vi "main.vi"() -> ()   [LabVIEW 2022 SP3]
uses:
  DataCluster.ctl
  a6309c79-5fe6-4af4-a42e-9fe127667a0f.vi
  b788d839-f62c-4f6b-a444-0fc034ee0148.vi
panel:
  in  "Delete":bool
  out "Progress":u8(slide)=100 scale=0.0..100.0
  in  "Download":bool
  out "Version":string="DL20 DG\nVersion 0.0.0.1"
  in  "Help":bool
  in  "File List":i32(listbox)=1
  out "Data Feed":string
  out "StatusString":string="Closing System"
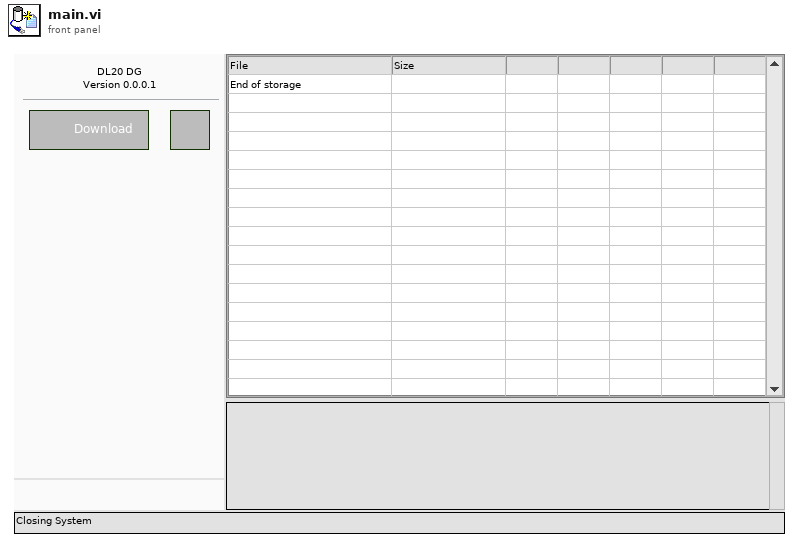
[diagram p1: front panel]
types:
  T1 = typedef "DataCluster.ctl" = cluster{"Core":cluster{"Current VI Reference":refnum<vi>, "Close Panel on Exit?":bool, "Exit":bool}, "Connections":cluster{"Arduino":cluster{"VISA":refnum<visa-resource-name>, "Data Feed":string, "Connected":bool}, "Ready":bool}, "Files":cluster{"Path":path, "Filename":string, "File List":i32, "Buffer":cluster{"Buffer":refnum<queue>, "Size":i32}, "Downloading":bool}}
  T2 = enum32{"Invalid", "Standard", "Closed", "Hidden", "Minimized", "Maximized"}
  T3 = enum32{"invalid app kind", "Development System", "Run Time System", "Student Edition", "Embedded LabVIEW", "Evaluation", "Custom"}
  T4 = cluster{"Arduino":cluster{"VISA":refnum<visa-resource-name>, "Data Feed":string, "Connected":bool}, "Ready":bool}
  T5 = enum8{"Enabled", "Disabled", "Disabled and Grayed Out"}
  T6 = cluster{"Current VI Reference":refnum<vi>, "Close Panel on Exit?":bool, "Exit":bool}
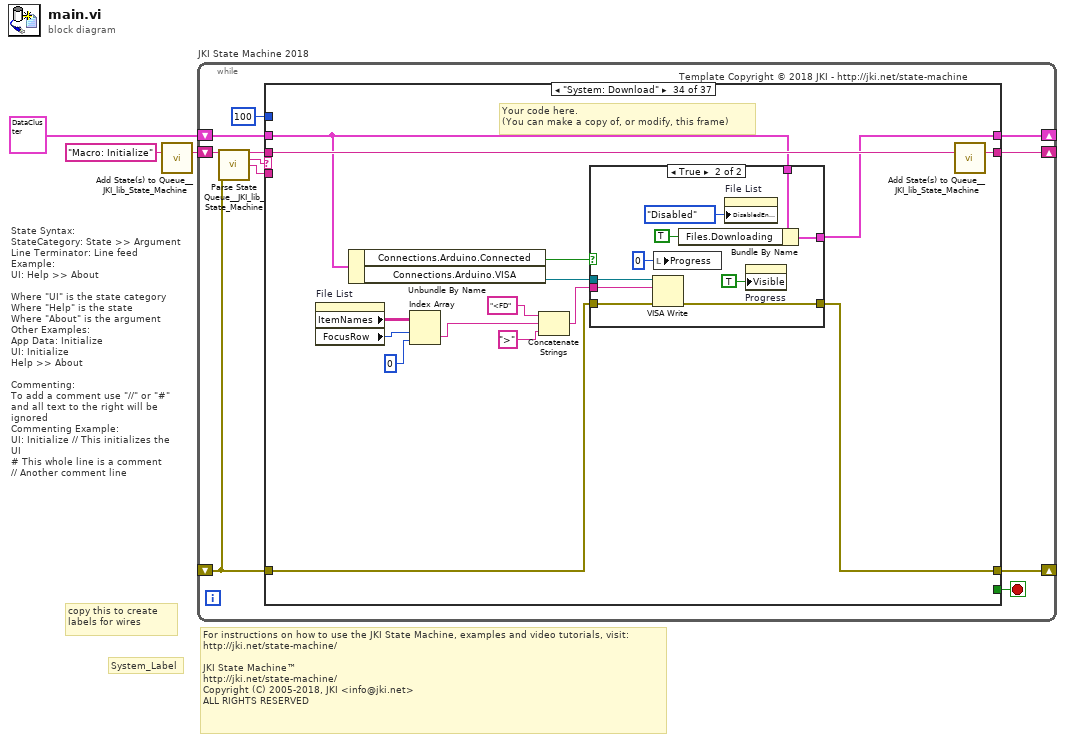
[diagram p0: block diagram]
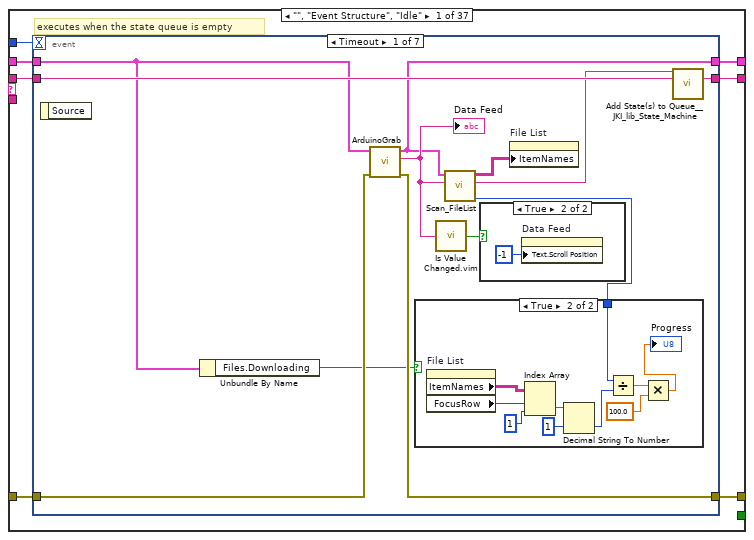
[diagram p2: hidden frame]
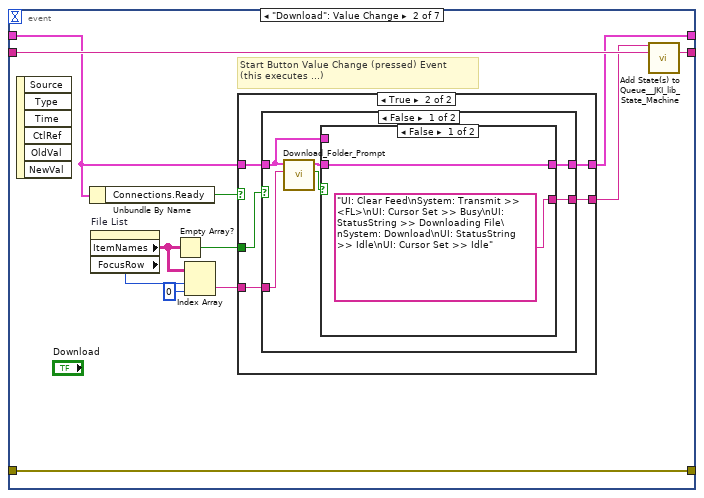
[diagram p5: hidden frame]
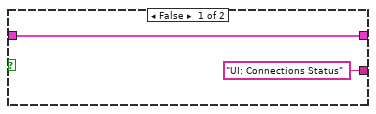
[diagram p6: hidden frame]
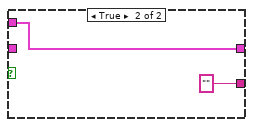
[diagram p7: hidden frame]
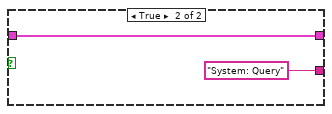
[diagram p8: hidden frame]
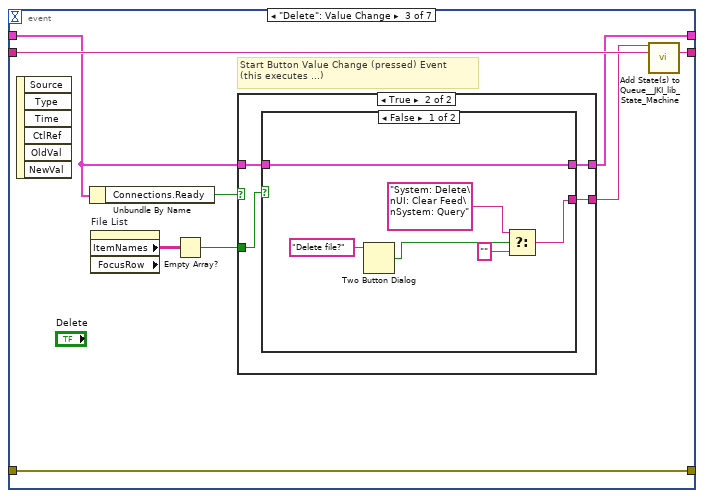
[diagram p9: hidden frame]
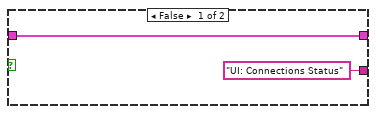
[diagram p10: hidden frame]
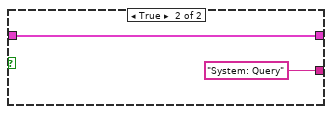
[diagram p11: hidden frame]
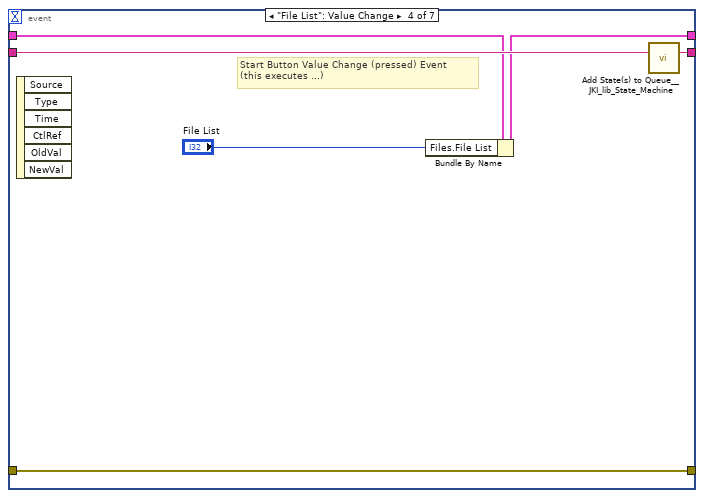
[diagram p12: hidden frame]
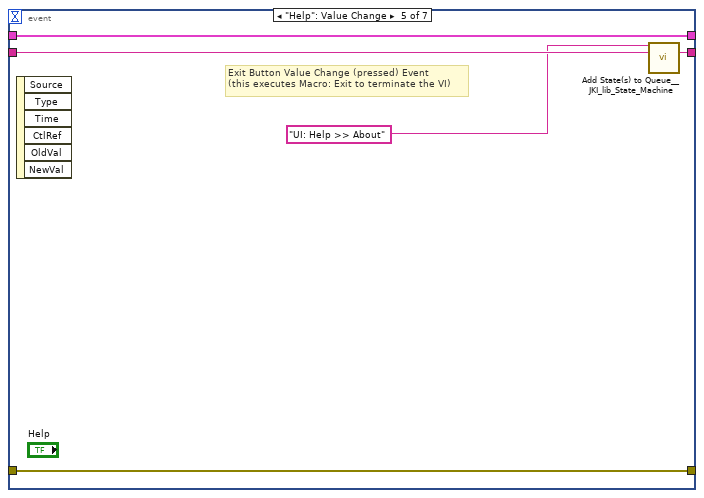
[diagram p13: hidden frame]
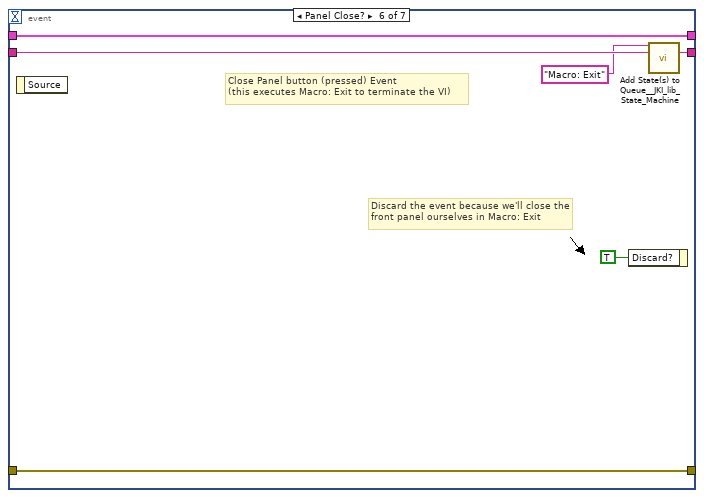
[diagram p14: hidden frame]
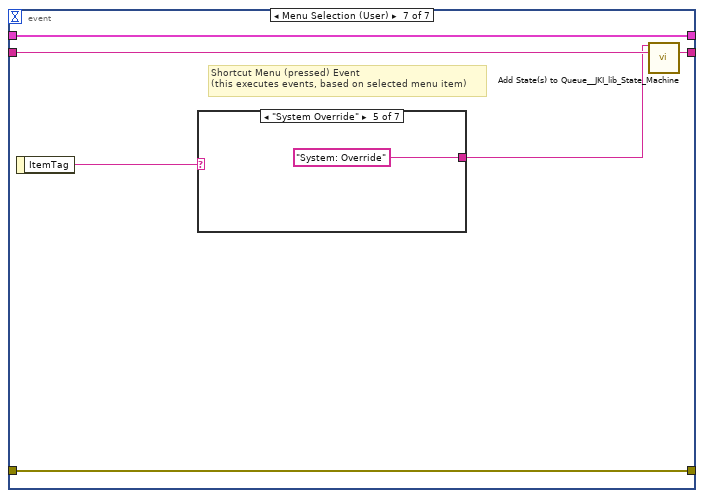
[diagram p15: hidden frame]
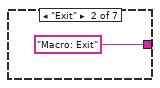
[diagram p17: hidden frame]
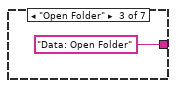
[diagram p18: hidden frame]
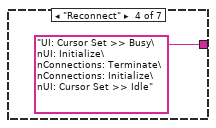
[diagram p19: hidden frame]
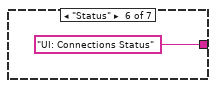
[diagram p20: hidden frame]
diagram:
  # "For instructions on how to use the JKI State Machine, examples and video tutorials, visit:\nhttp://jki.net/state-machine/\n\nJKI State Machine™\nhttp://jki.net/state-machine/\nCopyright (C) 2005-2018, JKI <info@jki.net>\nALL RIGHTS RESERVED"
  # "State Syntax:\nStateCategory: State >> Argument\nLine Terminator: Line feed\nExample:\nUI: Help >> About\n\nWhere \"UI\" is the state category\nWhere \"Help\" is the state\nWhere \"About\" is the argument\nOther Examples:\nApp Data: Initialize\nUI: Initialize\nHelp >> About\n\nCommenting:\nTo add a comment use \"//\" or \"#\" and all text to the right will be ignored\nCommenting Example:\nUI: Initialize // This initializes the UI\n# This whole line is a comment\n// Another comment line"
  # "copy this to create labels for wires"
  # "System_Label"
  n1 = call <vilib>:"Add State(s) to Queue__JKI_lib_State_Machine.vi"("State(s) in (\"\")"="Macro: Initialize") -> ("States Out"=w3:string)  [unwired: 14 in]
  n2 = while "JKI State Machine 2018" {
    shift-right: [w4] -> _
    shift-left: T1 {"Core"={"Current VI Reference"=refnum, "Close Panel on Exit?"=FALSE, "Exit"=FALSE}, "Connections"={"Arduino"={"VISA"="", "Data Feed"="", "Connected"=FALSE}, "Ready"=FALSE}, "Files"={"Path"=path "", "Filename"="", "File List"=0, "Buffer"={"Buffer"=refnum, "Size"=0}, "Downloading"=FALSE}} ("DataCluster") -> [w7]
    shift-right: [w10] -> _
    shift-left: _ -> [w5]
    shift-right: [w9] -> _
    shift-left: w3 -> [w11]
    stop <- w8 stop-if-true
    # "Template Copyright © 2018 JKI - http://jki.net/state-machine"
    n3 = call <vilib>:"Parse State Queue__JKI_lib_State_Machine.vi"("State Queue"=w11, "Error In (no error)"=w5) -> ("Remaining States"=w13:string, "Current State"=w14:string, "Arguments"=w12:string)  [unwired: 11 in]
    n4 = case shown="\"System: Download\"" w14 {
      selector: w14 -> [_ _ w132 _ _ _ _ _ _ _ _ _ _ _ _ _ _ _ _ _ _ _ _ _ _ _ _ _ _ _ _ _ _ _ _ _ _]
      tunnel: w13 -> [w21 w131 w136 w155 w161 w168 w172 w181 w188 w192 w199 w208 w212 w217 w225 w230 w238 w253 w265 w275 w285 w290 w295 w304 w313 w329 w340 w409 w414 w425 w429 w437 w450 w470 w498 w516 w520]
      tunnel: w12 -> [_ _ _ _ _ _ _ _ _ _ _ _ _ _ _ _ _ _ _ _ _ w286 w291 _ w309 w324 w334 _ _ _ _ w431 _ _ _ _ _]
      tunnel: w7 -> [w19 w128 w134 w148 w158 w164 w169 _ w185 w189 w196 w201 w209 w214 w221 w227 w234 w249 w262 w273 w283 w288 w293 w301 w311 w327 w336 w406 w411 w422 w426 w435 w448 w456 w483 w509 w517]
      tunnel: [w18 w129 w138 w152 errorcluster {"status"=FALSE, "code"=0, "source"=""} ("error out") w166 w170 w174 w182 w190 w193 w202 w210 w215 w222 w228 w231 w251 w263 w272 w282 w287 w292 w302 w310 w325 w337 w407 w412 w423 w427 w430 w444 w465 w493 w507 w518] -> w10
      tunnel: w5 -> [w17 w129 w137 w152 w157 w166 w170 w175 w184 w190 w194 w203 w210 w215 w223 w228 w232 w251 w263 w272 w282 w287 w292 w302 w310 w326 w338 w407 w412 w423 w427 w432 w445 w466 w494 w508 w518]
      tunnel: [w20 w130 w135 w154 w160 w167 w171 w180 w187 w191 w198 w207 w211 w216 w224 w229 w237 w252 w264 w274 w284 w289 w294 w303 w312 w328 w339 w408 w413 w424 w428 w436 w449 w469 w497 w515 w519] -> w9
      tunnel: [_ _ _ _ _ TRUE _ _ _ _ _ _ _ _ _ _ _ _ _ _ _ _ _ _ _ _ _ _ _ _ _ _ _ _ _ _ _] -> w8
      tunnel: [w16 w128 w134 w153 w158 w162 w169 w179 w185 w189 w196 w201 w209 w214 w220 w227 w233 w248 w262 w273 w281 w288 w293 w301 w311 w327 w336 w406 w411 w422 w426 w435 w448 w457 w483 w514 w517] -> w4
      tunnel: 100 ("Timeout") -> [w15 _ _ _ _ _ _ _ _ _ _ _ _ _ _ _ _ _ _ _ _ _ _ _ _ _ _ _ _ _ _ _ _ _ _ _ _]
      frame "", "Event Structure", "Idle" {
        # "executes when the state queue is empty"
        n5 = event shown="[0] Timeout" {
          selector: _ -> [_ _ _ _ _ _ _]
          dyn-events: _ -> [_ _ _ _ _ _ _]
          timeout: w15 -> [_ _ _ _ _ _ _]
          tunnel: w21 -> [w33 w56 w84 w104 w109 w115 w121]
          tunnel: [w32 w55 w83 w103 w108 w114 w120] -> w20
          tunnel: w19 -> [w25 w50 w78 w101 w106 w112 w118]
          tunnel: [w30 w54 w82 w102 w107 w113 w119] -> w18
          tunnel: w17 -> [w31 w54 w82 w102 w107 w113 w119]
          tunnel: [w22 w49 w77 w100 w106 w112 w118] -> w16
          event Timeout {
            n6 = event-data() -> ()  [unwired: 1 in, 1 out]
            n7 = Unbundle By Name(w25) -> ("Files.Downloading"=w24:bool)
            n8 = call "ArduinoGrab.vi"("error in (no error)"=w31, "DataCluster"=w25) -> ("error out"=w30:errorcluster, "read buffer out"=w23:string, "DataCluster out"=w22:T1)  [unwired: 6 in, 1 out]
            "Data Feed" <- w23
            n9 = call "Is Value Changed.vim"("value"=w23) -> ("changed or first call?"=w28:bool)
            n10 = call "Scan_FileList.vi"("Data Feed"=w23, "DataCluster"=w22) -> ("Downloaded bytes"=w27:i32, "state out"=w26:string, "Sorted Files"=w29:string[][])  [unwired: 7 in]
            n11 = case shown="True" w24 {
              tunnel: w27 -> [_ w35]
              frame False {
              }
              frame True {
                n12 = property on="File List" class="MCListbox (strict)"() -> ("ItemNames"=w43:string[][], "FocusRow"=w42:i32)  [unwired: 2 in, 2 out]
                n13 = Index Array(array=w43, index (row)=w42, index (col)=1 ("disabled index (col)")) -> (element=w40:string)
                n14 = Decimal String To Number(string=w40, offset=1) -> (number=w39:i32)  [unwired: 1 in, 1 out]
                n15 = Divide(x=w35, y=w39) -> (x/y=w38:dbl)
                n16 = Multiply(x=w38, y=100.0) -> (x*y=→"Progress":dbl)
              }
            }
            n17 = case shown="True" w28 {
              frame False {
              }
              frame True {
                n18 = property on="Data Feed" class="Str"("Text.Scroll Position"=-1) -> ()  [unwired: 2 in, 2 out]
              }
            }
            n19 = property on="File List" class="MCListbox (strict)"("ItemNames"=w29) -> ()  [unwired: 2 in, 2 out]
            n20 = call <vilib>:"Add State(s) to Queue__JKI_lib_State_Machine.vi"("State(s) in Front (\"\")"=w26, "State(s) in (\"\")"=w33) -> ("States Out"=w32:string)  [unwired: 13 in]
          }
          event "Download": Value Change {
            # "Start Button Value Change (pressed) Event\n(this executes ...)"
            n21 = event-data() -> ()  [unwired: 1 in, 6 out]
            n22 = Unbundle By Name(w50) -> ("Connections.Ready"=w52:bool)
            n23 = property on="File List" class="MCListbox (strict)"() -> ("ItemNames"=w48:string[][], "FocusRow"=w47:i32)  [unwired: 2 in, 2 out]
            n24 = Empty Array?(array=w48) -> (empty?=w51:bool)
            n25 = Index Array(array=w48, index (row)=w47, index (col)=0 ("disabled index (col)")) -> (element=w45:string)
            n26 = case shown="True" w52 {
              tunnel: ["UI: Connections Status" ("State(s) in Front (\"\")") w63] -> w53
              tunnel: w51 -> [_ w62]
              tunnel: w50 -> [w57 w61]
              tunnel: [w57 w60] -> w49
              tunnel: w45 -> [_ w59]
              frame False {
              }
              frame True {
                n27 = case shown="False" w62 {
                  tunnel: [w69 "System: Query" ("State(s) in Front (\"\")")] -> w63
                  tunnel: w61 -> [w65 w74]
                  tunnel: [w66 w74] -> w60
                  tunnel: w59 -> [w64 _]
                  frame False {
                    n28 = call "Download_Folder_Prompt.vi"("default name"=w64, "DataCluster"=w65) -> ("cancled?"=w68:bool, "DataCluster out"=w67:T1)  [unwired: 8 in]
                    n29 = case shown="False" w68 {
                      tunnel: ["UI: Clear Feed\nSystem: Transmit >> <FL>\nUI: Cursor Set >> Busy\nUI: StatusString >> Downloading File\nSystem: Download\nUI: StatusString >> Idle\nUI: Cursor Set >> Idle" ("State(s) in Front (\"\")") "" ("State(s) in Front (\"\")")] -> w69
                      tunnel: [w70 w73] -> w66
                      tunnel: w67 -> [w70 _]
                      tunnel: w65 -> [_ w73]
                      frame False {
                      }
                      frame True {
                      }
                    }
                  }
                  frame True {
                  }
                }
              }
            }
            n30 = call <vilib>:"Add State(s) to Queue__JKI_lib_State_Machine.vi"("State(s) in Front (\"\")"=w53, "State(s) in (\"\")"=w56) -> ("States Out"=w55:string)  [unwired: 13 in]
          }
          event "Delete": Value Change {
            # "Start Button Value Change (pressed) Event\n(this executes ...)"
            n31 = event-data() -> ()  [unwired: 1 in, 6 out]
            n32 = Unbundle By Name(w78) -> ("Connections.Ready"=w80:bool)
            n33 = property on="File List" class="MCListbox (strict)" props=["ItemNames", "FocusRow"]() -> ("ItemNames"=w76:string[][])  [unwired: 2 in, 3 out]
            n34 = Empty Array?(array=w76) -> (empty?=w79:bool)
            n35 = case shown="True" w80 {
              tunnel: ["UI: Connections Status" ("State(s) in Front (\"\")") w90] -> w81
              tunnel: w79 -> [_ w89]
              tunnel: w78 -> [w85 w88]
              tunnel: [w85 w87] -> w77
              frame False {
              }
              frame True {
                n36 = case shown="False" w89 {
                  tunnel: [w92 "System: Query" ("State(s) in Front (\"\")")] -> w90
                  tunnel: w88 -> [w96 w97]
                  tunnel: [w96 w97] -> w87
                  frame False {
                    n37 = Two Button Dialog(message="Delete file?") -> (T button?=w94:bool)  [unwired: 2 in]
                    n38 = Select(t="System: Delete\nUI: Clear Feed\nSystem: Query" ("State(s) in Front (\"\")"), s=w94, f="") -> (s? t:f=w92:string)
                  }
                  frame True {
                  }
                }
              }
            }
            n39 = call <vilib>:"Add State(s) to Queue__JKI_lib_State_Machine.vi"("State(s) in Front (\"\")"=w81, "State(s) in (\"\")"=w84) -> ("States Out"=w83:string)  [unwired: 13 in]
          }
          event "File List": Value Change {
            # "Start Button Value Change (pressed) Event\n(this executes ...)"
            n40 = event-data() -> ()  [unwired: 1 in, 6 out]
            n41 = Bundle By Name(cluster=w101, "Files.File List"="File List") -> (w100:T1)
            n42 = call <vilib>:"Add State(s) to Queue__JKI_lib_State_Machine.vi"("State(s) in (\"\")"=w104) -> ("States Out"=w103:string)  [unwired: 14 in]
          }
          event "Help": Value Change {
            # "Exit Button Value Change (pressed) Event\n(this executes Macro: Exit to terminate the VI)"
            n43 = event-data() -> ()  [unwired: 1 in, 6 out]
            n44 = call <vilib>:"Add State(s) to Queue__JKI_lib_State_Machine.vi"("State(s) in Front (\"\")"="UI: Help >> About" ("State(s) in Front (\"\")"), "State(s) in (\"\")"=w109) -> ("States Out"=w108:string)  [unwired: 13 in]
          }
          event Panel Close? {
            # "Discard the event because we'll close the front panel ourselves in Macro: Exit"
            # "Close Panel button (pressed) Event\n(this executes Macro: Exit to terminate the VI)"
            n45 = event-data() -> ()  [unwired: 1 in, 1 out]
            n46 = event-data("Discard?"=TRUE) -> ()  [unwired: 1 in, 1 out]
            n47 = call <vilib>:"Add State(s) to Queue__JKI_lib_State_Machine.vi"("State(s) in Front (\"\")"="Macro: Exit", "State(s) in (\"\")"=w115) -> ("States Out"=w114:string)  [unwired: 13 in]
          }
          event Menu Selection (User) {
            # "Shortcut Menu (pressed) Event\n(this executes events, based on selected menu item)"
            n48 = event-data() -> ("ItemTag"=w117:string)  [unwired: 1 in]
            n49 = case shown="\"System Override\"" w117 {
              tunnel: [_ "Macro: Exit" "Data: Open Folder" "UI: Cursor Set >> Busy\nUI: Initialize\nConnections: Terminate\nConnections: Initialize\nUI: Cursor Set >> Idle" "System: Override" "UI: Connections Status" "UI: Clear Feed\nSystem: Query"] -> w116
              frame "False", Default {
              }
              frame "Exit" {
              }
              frame "Open Folder" {
              }
              frame "Reconnect" {
              }
              frame "System Override" {
              }
              frame "Status" {
              }
              frame "Requery" {
              }
            }
            n50 = call <vilib>:"Add State(s) to Queue__JKI_lib_State_Machine.vi"("State(s) in Front (\"\")"=w116, "State(s) in (\"\")"=w121) -> ("States Out"=w120:string)  [unwired: 13 in]
          }
        }
      }
      frame "---------- Core ----------" {
        # "Do not put any code in this frame.\n(it is a separator no-op)"
        n51 = call <vilib>:"Add State(s) to Queue__JKI_lib_State_Machine.vi"("State(s) in (\"\")"=w131) -> ("States Out"=w130:string)  [unwired: 14 in]
      }
      frame Default {
        w141 = 42 items=["No error", "Argument error", "Memory is full", "Out of zone", "End of file", "File already open", "Generic file I/O error", "File not found", "File permission error", "Disk is full", "Duplicate path", "Too many files open", "System feature not enabled", "Resource file not found", "Cannot add resource", "Resource not found", "Image not found", "Image memory error", "Pen does not exist", "Config type invalid", "Config token not found", "Config parse error", "Config memory error", "Bad external code format", "Bad external code offset", "External code not present", "Null window", "Destroy window error", "Null menu", "Print aborted", "Bad print record", "Print driver error", "Windows error during printing", "Memory error during printing", "Print dialog error", "Generic print error", "Invalid device refnum", "Device not found", "Device parameter error", "Device unit error", "Cannot open device", "Device call aborted", "Generic error", "Cancelled by user", "Object ID too low", "Object ID too high", "Object not in heap", "Unknown heap", "Unknown object (invalid DefProc)", "Unknown object (DefProc not in table)", "Message out of range", "Invalid (null) method", "Unknown message", "Manager call not supported", "Bad address", "Network operation in progress", "Network operation timed out", "Connection is busy", "Network attribute not supported", "Network error", "Address in use", "System out of memory", "Connection aborted", "Connection refused", "Not connected", "Already connected", "Connection closed", "Initialization error (interapplication manager)", "Bad occurrence", "Wait on unbound occurrence handler", "Occurrence queue overflow", "Datalog type conflict", "Unused", "Unrecognized type (interapplication manager)", "Memory corrupt", "Failed to make temporary DLL", "Old CIN version", "Drag socket not found", "Failed to load drop-object", "Failed to register OLE object", "Failed to release OLE object", "Format specifier type mismatch", "Unknown format specifier", "Too few format specifiers", "Too many format specifiers", "Scan failed", "Newer CIN version", "Error converting to variant", "Runtime menu error", "Password tampered", "Variant attribute not found", "Incompatible variant data type", "Event data is not available", "Event Store is not present", "Occurrence is not found", "Event Queue is not created", "Event info is not available", "Refnum passed is NULL", "Error retrieving Class GUID", "Error retrieving CoClass GUID", "Error retrieving TypeLib GUID.", "Bad built application magic bytes.", "Specific driver is different from the specific driver associated with the Logical Name.", "There is no session opened to the class driver.", "Max Error", "MAX - Error with config objects", "MAX - Error loading configuration", "MAX - Group not supported"]
        # "Current State"
        # "Do not delete, rename, or modify this frame.\n(this is used to capture unhandled states and typos)"
        # "Handle mistyped state name (developer tool)"
        n52 = Format Into String(format string="Software Exception: Unhandled State \"%s\"." ("message"), error in=w137, w132) -> (resulting string=w140:string, error out=w139:errorcluster)  [unwired: 1 in]
        n53 = call <vilib>:"Error Cluster From Error Code.vi"("show call chain? (False)"=TRUE, "error in (no error)"=w139, "error message (\"\")"=w140, "error code (0)"=w141) -> ("error out"=w138:errorcluster)  [unwired: 5 in]
        n54 = call <vilib>:"Add State(s) to Queue__JKI_lib_State_Machine.vi"("State(s) in (\"\")"=w136) -> ("States Out"=w135:string)  [unwired: 14 in]
      }
      frame "Initialize Core Data" {
        # "Do not delete, rename, or modify this frame.\n(this is used to determine panel behavior on exit)"
        # "originally closed?"
        # "exe?"
        # "If panel starts closed or is an EXE, then close it when we exit"
        n55 = property class="VI"() -> ("FP.State"=w145:T2)  [unwired: 2 in, 2 out]
        n56 = property class="App"() -> ("App.Kind"=w151:T3)  [unwired: 2 in, 2 out]
        n57 = control-ref of="Current VI Reference"() -> (w146:refnum<vi>)
        n58 = Equal?(x=w145, y=T2."Closed" ("Front Panel Window:State")) -> (x = y?=w143:bool)
        n59 = Equal?(x=w151, y=T3."Run Time System" ("Application:Kind")) -> (x = y?=w149:bool)
        n60 = Or(x=w143, y=w149) -> (x .or. y?=w147:bool)
        n61 = Bundle By Name(cluster=w148, "Core.Current VI Reference"=w146, "Core.Close Panel on Exit?"=w147) -> (w153:T1)
        n62 = call <vilib>:"Add State(s) to Queue__JKI_lib_State_Machine.vi"("State(s) in (\"\")"=w155) -> ("States Out"=w154:string)  [unwired: 14 in]
      }
      frame "Error Handler" {
        # "Unhandled Error -- Display it"
        # "Handle any errors here.\nYou can also output any states to clean-up after errors occur"
        # "Clear error"
        n63 = call <vilib>:"General Error Handler.vi"("error in (no error)"=w157) -> ()  [unwired: 10 in, 5 out]
        n64 = call <vilib>:"Add State(s) to Queue__JKI_lib_State_Machine.vi"("State(s) in Front (\"\")"="/* Post Error States", "State(s) in (\"\")"=w161) -> ("States Out"=w160:string)  [unwired: 13 in]
      }
      frame "Exit" {
        # "Do not put any code in this frame.\n(No errors that occur here will be handled.)"
        n65 = Bundle By Name(cluster=w164, "Core.Exit"=TRUE) -> (w162:T1)
        n66 = call <vilib>:"Add State(s) to Queue__JKI_lib_State_Machine.vi"("State(s) in (\"\")"=w168) -> ("States Out"=w167:string)  [unwired: 14 in]
      }
      frame "---------- Data ----------" {
        # "Do not put any code in this frame.\n(It is a separator no-op. You can make a copy of this frame to create a new Data frame)"
        n67 = call <vilib>:"Add State(s) to Queue__JKI_lib_State_Machine.vi"("State(s) in (\"\")"=w172) -> ("States Out"=w171:string)  [unwired: 14 in]
      }
      frame "Data: Initialize" {
        w178 = T6 {"Current VI Reference"=refnum, "Close Panel on Exit?"=FALSE, "Exit"=FALSE}  # Core
        # "Initialize the shift-register data, here.\n(data names are defined by what you wire into the bundle function)"
        n68 = call "Settings_Load.vi"("error in"=w175) -> ("error out"=w176:errorcluster, "DataCluster out"=w177:T1)  [unwired: 9 in]
        n69 = call "Settings_Save.vi"("error in"=w176, "DataCluster"=w177) -> ("error out"=w174:errorcluster)  [unwired: 9 in]
        n70 = Bundle By Name(cluster=w177, "Core"=w178, "Connections"=T4 {"Arduino"={"VISA"="", "Data Feed"="", "Connected"=FALSE}, "Ready"=FALSE}) -> (w179:T1)
        n71 = call <vilib>:"Add State(s) to Queue__JKI_lib_State_Machine.vi"("State(s) in (\"\")"=w181) -> ("States Out"=w180:string)  [unwired: 14 in]
      }
      frame "Data: Cleanup" {
        # "Cleanup any data and references, here.\n(this is called automatically, by the Macro: Exit)"
        n72 = Unbundle By Name(w185) -> ("Core.Current VI Reference"=w186:refnum<vi>)
        n73 = call "Settings_Save.vi"("error in"=w184, "DataCluster"=w185) -> ("error out"=w183:errorcluster)  [unwired: 9 in]
        n74 = Close Reference(reference=w186, error in (no error)=w183) -> (error out=w182:errorcluster)
        n75 = call <vilib>:"Add State(s) to Queue__JKI_lib_State_Machine.vi"("State(s) in (\"\")"=w188) -> ("States Out"=w187:string)  [unwired: 14 in]
      }
      frame "Data: Options" {
        # "Access Data Setup here.\n(this is called automatically, by the Settings Event Run time menu)"
        n76 = call <vilib>:"Add State(s) to Queue__JKI_lib_State_Machine.vi"("State(s) in (\"\")"=w192) -> ("States Out"=w191:string)  [unwired: 14 in]
      }
      frame "Data: Files Unlock" {
        # "Unluck Data filehere.\n(this is called automatically, by the Settings Event Run time menu)"
        n77 = Unbundle By Name(w196) -> ("Files.Path"=w195:path)
        n78 = Set Permissions(7:i16 448 ("permissions"), 8:w194, 11:w195) -> (0:w193:errorcluster)  [unwired: 2 in, 1 out]
        n79 = call <vilib>:"Add State(s) to Queue__JKI_lib_State_Machine.vi"("State(s) in (\"\")"=w199) -> ("States Out"=w198:string)  [unwired: 14 in]
      }
      frame "Data: Open Folder" {
        # "Access Data Setup here.\n(this is called automatically, by the Settings Event Run time menu)"
        n80 = Unbundle By Name(w201) -> ("Files.Path"=w200:path)
        n81 = Format Into String(format string="cmd /c explorer.exe \"%s\"", w200) -> (resulting string=w205:string)  [unwired: 2 in, 1 out]
        n82 = call <vilib>:"System Exec.vi"("run minimized? (F)"=TRUE, "error in (no error)"=w203, "command line"=w205) -> ("error out"=w202:errorcluster)  [unwired: 5 in, 3 out]
        n83 = call <vilib>:"Add State(s) to Queue__JKI_lib_State_Machine.vi"("State(s) in (\"\")"=w208) -> ("States Out"=w207:string)  [unwired: 14 in]
      }
      frame "---------- Connections ----------" {
        # "Do not put any code in this frame.\n(It is a separator no-op. You can make a copy of this frame to create a new Data frame)"
        n84 = call <vilib>:"Add State(s) to Queue__JKI_lib_State_Machine.vi"("State(s) in (\"\")"=w212) -> ("States Out"=w211:string)  [unwired: 14 in]
      }
      frame "Connections: Initialize" {
        # "Initialize the System Connections, here.\n(this is called automatically, by the Macro: Init)"
        n85 = call <vilib>:"Add State(s) to Queue__JKI_lib_State_Machine.vi"("State(s) in Front (\"\")"="UI: StatusString >> Connecting to System\nConnections: Initialize Arduino\nUI: StatusString >> Validating Connections\nConnections: Status" ("State(s) in Front (\"\")"), "State(s) in (\"\")"=w217) -> ("States Out"=w216:string)  [unwired: 13 in]
      }
      frame "Connections: Initialize Arduino" {
        # "Initialize the System Connections, here.\n(this is called automatically, by the Macro: Init)"
        n86 = call "ConnectionArduino.vi"("error in"=w223) -> ("error out"=w222:errorcluster, 2:"Arduino"=w218:bool, 3:"Arduino"=w219:refnum<visa-resource-name>)  [unwired: 8 in]
        n87 = Bundle By Name(cluster=w221, "Connections.Arduino.VISA"=w219, "Connections.Arduino.Connected"=w218) -> (w220:T1)
        n88 = call <vilib>:"Add State(s) to Queue__JKI_lib_State_Machine.vi"("State(s) in (\"\")"=w225) -> ("States Out"=w224:string)  [unwired: 14 in]
      }
      frame "Connections: Terminate" {
        # "Terminate connections"
        # "Terminate the System Connections, here.\n(this is called automatically, by the Macro: Exit)"
        n89 = call <vilib>:"Add State(s) to Queue__JKI_lib_State_Machine.vi"("State(s) in Front (\"\")"="UI: StatusString >> Terminating System Connection\nConnections: Terminate Arduino" ("State(s) in Front (\"\")"), "State(s) in (\"\")"=w230) -> ("States Out"=w229:string)  [unwired: 13 in]
      }
      frame "Connections: Terminate Arduino" {
        # "Terminate connection to Arduino"
        # "Terminate the System Connections, here.\n(this is called automatically, by the Macro: Exit)"
        n90 = Unbundle By Name(w234) -> ("Connections.Arduino.VISA"=w235:refnum<visa-resource-name>, "Connections.Arduino.Connected"=w236:bool)
        n91 = case shown="True" w236 {
          tunnel: w235 -> [_ w241]
          tunnel: w234 -> [w240 w246]
          tunnel: [w240 w244] -> w233
          tunnel: w232 -> [w239 w243]
          tunnel: [w239 w242] -> w231
          frame False {
          }
          frame True {
            n92 = VISA Close(VISA resource name=w241, error in (no error)=w243) -> (error out=w242:errorcluster)
            n93 = Bundle By Name(cluster=w246, "Connections.Arduino.Connected"=FALSE ("Connections.cDAQ.Connected")) -> (w244:T1)
          }
        }
        n94 = call <vilib>:"Add State(s) to Queue__JKI_lib_State_Machine.vi"("State(s) in (\"\")"=w238) -> ("States Out"=w237:string)  [unwired: 14 in]
      }
      frame "Connections: Status" {
        # "Checks Connection Status , here.\n(this is called automatically, by the Connections: Initialize)"
        n95 = Unbundle By Name(w249) -> ("Connections.Arduino.Connected"=w247:bool)
        n96 = case shown="False" w247 {
          selector: w247 -> [w254 w259]
          tunnel: ["UI: Start Button >> Error\nUI: StatusString >> Connection Error!" "UI: Start Button >> Default\nUI: StatusString >> Idle"] -> w250
          tunnel: w249 -> [w256 w260]
          tunnel: [w255 w258] -> w248
          frame False {
            n97 = Bundle By Name(cluster=w256, "Connections.Ready"=w254) -> (w255:T1)
          }
          frame True {
            n98 = Bundle By Name(cluster=w260, "Connections.Ready"=w259) -> (w258:T1)
          }
        }
        n99 = call <vilib>:"Add State(s) to Queue__JKI_lib_State_Machine.vi"("State(s) in Front (\"\")"=w250, "State(s) in (\"\")"=w253) -> ("States Out"=w252:string)  [unwired: 13 in]
      }
      frame "---------- UI ----------" {
        # "Do not put any code in this frame.\n(It is a separator no-op. You can make a copy of this frame to create a new UI frame)"
        n100 = call <vilib>:"Add State(s) to Queue__JKI_lib_State_Machine.vi"("State(s) in (\"\")"=w265) -> ("States Out"=w264:string)  [unwired: 14 in]
      }
      frame "UI: Initialize" {
        # "Initialize the User Interface, here.\n(this is called automatically, by the Macro: Init)"
        n101 = for {
          N: 50 -> [_]
          i -> [w278]
          n102 = Bundle(w278, 1) -> (w279:cluster{i32, i32})  [unwired: 1 in]
          n103 = property on="File List" class="MCListbox (strict)"("ActiveCell"=w279, "Justify"=enum16{"Left", "Center", "Right"}."Right" ("Active Cell:Cell Justification")) -> ()  [unwired: 2 in, 2 out]
        }
        n104 = property on="File List" class="MCListbox (strict)"("ItemNames"=string[][] [] ("Item Names")) -> ()  [unwired: 2 in, 2 out]
        n105 = call "Read Exe Version.vi"() -> ("String"=→"Version":string)  [unwired: 10 in, 1 out]
        n106 = property on="Progress" class="Slide (strict)"("Visible"=FALSE) -> ()  [unwired: 2 in, 2 out]
        n107 = property on="File List" class="MCListbox (strict)"("DisabledEnum"=T5."Enabled" ("Disabled")) -> ()  [unwired: 2 in, 2 out]
        n108 = call <vilib>:"Add State(s) to Queue__JKI_lib_State_Machine.vi"("State(s) in Front (\"\")"="UI: Clear Feed" ("State(s) in Front (\"\")"), "State(s) in (\"\")"=w275) -> ("States Out"=w274:string)  [unwired: 13 in]
      }
      frame "UI: Clear Feed" {
        w280 = "" ("Data Feed")
        # "Initialize the User Interface, here.\n(this is called automatically, by the Macro: Init)"
        n109 = Bundle By Name(cluster=w283, "Connections.Arduino.Data Feed"=w280) -> (w281:T1)
        n110 = local write "Data Feed"(w280) -> ()
        n111 = call <vilib>:"Add State(s) to Queue__JKI_lib_State_Machine.vi"("State(s) in (\"\")"=w285) -> ("States Out"=w284:string)  [unwired: 14 in]
      }
      frame "UI: StatusString" {
        # "Argument"
        # "Set Status String here\n(this is called takes argument and applies to Status String)"
        n112 = call <vilib>:"Add State(s) to Queue__JKI_lib_State_Machine.vi"("State(s) in (\"\")"=w290) -> ("States Out"=w289:string)  [unwired: 14 in]
        "StatusString" <- w286
      }
      frame "UI: Help" {
        # "Argument"
        # "Set Status String here\n(this is called takes argument and applies to Status String)"
        n113 = case shown="\"About\"" w291 {
          frame "False", Default {
          }
          frame "About" {
            n114 = call "Read Exe Version.vi"() -> ("String"=w296:string)  [unwired: 10 in, 1 out]
            n115 = Concatenate Strings("Drill Logger Data Grab\n\n" ("message"), w296) -> (w297:string)
            n116 = One Button Dialog(message=w297) -> ()  [unwired: 1 in, 1 out]
          }
        }
        n117 = call <vilib>:"Add State(s) to Queue__JKI_lib_State_Machine.vi"("State(s) in (\"\")"=w295) -> ("States Out"=w294:string)  [unwired: 14 in]
      }
      frame "UI: Connections Status" {
        # "Set Status String here\n(this is called takes argument and applies to Status String)"
        n118 = Unbundle By Name(w301) -> ("Connections.Arduino.Connected"=w300:bool)
        n119 = call "ConnectionStatus.vi"("Connection Status"=w300) -> ("String"=w299:string)  [unwired: 9 in, 1 out]
        n120 = call <vilib>:"Add State(s) to Queue__JKI_lib_State_Machine.vi"("State(s) in Front (\"\")"=w299, "State(s) in (\"\")"=w304) -> ("States Out"=w303:string)  [unwired: 13 in]
      }
      frame "UI: Start Button" {
        # "Argument"
        # "Set Status String here\n(this is called takes argument and applies to Status String)"
        n121 = case shown="\"Connecting\"" w309 {
          tunnel: [w314 cluster{u32, u32}[] [{1985280, 12369084}, {4367360, 4367360}, {8388608, 16711681}, {1985280, 1985280}, {1985280, 4367360}, {8388608, 16711681}] ("Colors [4]") w321] -> w306
          tunnel: [string[] ["  Error", "  Error", "  Error", "  Error"] ("Strings [4]") string[] ["Download", "Download", "Download", "Download"] ("Strings [4]") string[] ["Connecting", "Connecting", "Connecting", "Connecting"] ("Strings [4]")] -> w308
          tunnel: [T5."Enabled" ("Disabled") T5."Enabled" ("Disabled") T5."Disabled" ("Disabled")] -> w307
          tunnel: [w314 cluster{u32, u32}[] [{1985280, 12369084}, {8388608, 16711681}, {8388608, 16711681}, {8388608, 8388608}, {8388608, 8388608}, {8388608, 16711681}] ("Colors [4]") w321] -> w305
          frame "Error" {
            w314 = cluster{u32, u32}[] [{8388608, 8388608}, {4367360, 4367360}, {9342611, 9342611}, {6710891, 6710891}, {16711681, 16711680}, {16711681, 16711680}] ("Colors [4]")
          }
          frame "Default", Default {
          }
          frame "Connecting" {
            w321 = cluster{u32, u32}[] [{9342611, 9342611}, {4367360, 4367360}, {9342611, 9342611}, {6710891, 6710891}, {9342611, 9342611}, {9342611, 9342611}] ("Colors [4]")
          }
        }
        n122 = property on="Download" class="Bool"("Colors [4]"=w306, "Strings [4]"=w308, "DisabledEnum"=w307) -> ()  [unwired: 2 in, 2 out]
        n123 = property on="Delete" class="Bool"("Colors [4]"=w305, "DisabledEnum"=w307) -> ()  [unwired: 2 in, 2 out]
        n124 = call <vilib>:"Add State(s) to Queue__JKI_lib_State_Machine.vi"("State(s) in (\"\")"=w313) -> ("States Out"=w312:string)  [unwired: 14 in]
      }
      frame "UI: Cursor Set" {
        # "Argument"
        # "Set and Unset Cursor Busy.\n(Usage: \"UI: Cursor Set >> Busy|Idle\")"
        n125 = case shown="\"Idle\", Default" w324 {
          tunnel: w326 -> [w331 w333]
          tunnel: [w330 w332] -> w325
          frame "Idle", Default {
            n126 = call <vilib>:"Unset Busy.vi"("error in (no error)"=w331) -> ("error out"=w330:errorcluster)  [unwired: 10 in]
          }
          frame "Busy" {
            n127 = call <vilib>:"Set Busy.vi"("error in (no error)"=w333) -> ("error out"=w332:errorcluster)  [unwired: 9 in, 1 out]
          }
        }
        n128 = call <vilib>:"Add State(s) to Queue__JKI_lib_State_Machine.vi"("State(s) in (\"\")"=w329) -> ("States Out"=w328:string)  [unwired: 14 in]
      }
      frame "UI: Front Panel State" {
        # "Argument"
        # "Set Front Panel Open or Closed\n(Usage: \"UI: Front Panel State >> Open|Close\")"
        n129 = Unbundle By Name(w336) -> ("Core.Current VI Reference"=w335:refnum<vi>)
        n130 = case shown="\"Minimize\", \"Minimized\"" w334 {
          tunnel: w338 -> [w346 w361 w372 w385 w398]
          tunnel: [w348 w362 w374 w387 w400] -> w337
          tunnel: w335 -> [w347 w359 w373 w386 w399]
          frame "Open", "Standard", Default {
            w341 = T2."Standard" ("State")
            n131 = property class="VI"(reference=w347, error in=w346) -> (reference out=w344:refnum<vi>, error out=w345:errorcluster, "FP.State"=w343:T2)
            n132 = Not Equal?(x=w343, y=w341) -> (x != y?=w342:bool)
            n133 = case shown="True" w342 {
              tunnel: [w352 w354] -> w348
              tunnel: w345 -> [w351 w354]
              tunnel: w344 -> [w350 _]
              tunnel: w341 -> [w349 _]
              frame True {
                n134 = invoke class="VI" method="FP.Open"(reference=w350, error in=w351, "Activate"=TRUE, "State"=w349) -> (error out=w352:errorcluster)  [unwired: 1 in, 4 out]
              }
              frame False {
              }
            }
          }
          frame "Close", "Closed" {
            n135 = property class="VI"(reference=w359, error in=w361) -> (reference out=w358:refnum<vi>, error out=w360:errorcluster, "FP.State"=w356:T2)
            n136 = Not Equal?(x=w356, y=T2."Closed" ("Front Panel Window:State")) -> (x != y?=w355:bool)
            n137 = case shown="True" w355 {
              tunnel: [w363 w366] -> w362
              tunnel: w360 -> [w363 w365]
              tunnel: w358 -> [_ w364]
              frame False {
              }
              frame True {
                n138 = invoke class="VI" method="FP.Close"(reference=w364, error in=w365) -> (error out=w366:errorcluster)  [unwired: 1 in, 2 out]
              }
            }
          }
          frame "Hidden", "Hide" {
            w367 = T2."Hidden" ("State")
            n139 = property class="VI"(reference=w373, error in=w372) -> (reference out=w370:refnum<vi>, error out=w371:errorcluster, "FP.State"=w369:T2)
            n140 = Not Equal?(x=w369, y=w367) -> (x != y?=w368:bool)
            n141 = case shown="True" w368 {
              tunnel: [w378 w379] -> w374
              tunnel: w371 -> [w377 w379]
              tunnel: w370 -> [w376 _]
              tunnel: w367 -> [w375 _]
              frame True {
                n142 = invoke class="VI" method="FP.Open"(reference=w376, error in=w377, "State"=w375) -> (error out=w378:errorcluster)  [unwired: 2 in, 4 out]
              }
              frame False {
              }
            }
          }
          frame "Minimize", "Minimized" {
            w380 = T2."Minimized" ("State")
            n143 = property class="VI"(reference=w386, error in=w385) -> (reference out=w383:refnum<vi>, error out=w384:errorcluster, "FP.State"=w382:T2)
            n144 = Not Equal?(x=w382, y=w380) -> (x != y?=w381:bool)
            n145 = case shown="True" w381 {
              tunnel: [w391 w392] -> w387
              tunnel: w384 -> [w390 w392]
              tunnel: w383 -> [w389 _]
              tunnel: w380 -> [w388 _]
              frame True {
                n146 = invoke class="VI" method="FP.Open"(reference=w389, error in=w390, "State"=w388) -> (error out=w391:errorcluster)  [unwired: 2 in, 4 out]
              }
              frame False {
              }
            }
          }
          frame "Maximize", "Maximized" {
            w393 = T2."Maximized" ("State")
            n147 = property class="VI"(reference=w399, error in=w398) -> (reference out=w396:refnum<vi>, error out=w397:errorcluster, "FP.State"=w395:T2)
            n148 = Not Equal?(x=w395, y=w393) -> (x != y?=w394:bool)
            n149 = case shown="True" w394 {
              tunnel: [w404 w405] -> w400
              tunnel: w397 -> [w403 w405]
              tunnel: w396 -> [w402 _]
              tunnel: w393 -> [w401 _]
              frame True {
                n150 = invoke class="VI" method="FP.Open"(reference=w402, error in=w403, "State"=w401) -> (error out=w404:errorcluster)  [unwired: 2 in, 4 out]
              }
              frame False {
              }
            }
          }
        }
        n151 = call <vilib>:"Add State(s) to Queue__JKI_lib_State_Machine.vi"("State(s) in (\"\")"=w340) -> ("States Out"=w339:string)  [unwired: 14 in]
      }
      frame "---------- Macro ----------" {
        # "Do not put any code in this frame.\n(It is a separator no-op. You can make a copy of this frame to create a new Macro frame)"
        n152 = call <vilib>:"Add State(s) to Queue__JKI_lib_State_Machine.vi"("State(s) in (\"\")"=w409) -> ("States Out"=w408:string)  [unwired: 14 in]
      }
      frame "Macro: Initialize" {
        w410 = "UI: StatusString >> Initializing...\nUI: Cursor Set >> Busy\nUI: Start Button >> Connecting\nUI: StatusString >> Initializing Data\nData: Initialize\nUI: StatusString >> Initializing Core Data\nInitialize Core Data\nUI: StatusString >> Initializing User Interface\nUI: Initialize\nUI: StatusString >> Initializing Connections\nConnections: Initialize\nUI: StatusString >> Query Data\nSystem: Query\nConnections: Status\nUI: Front Panel State >> Open\nUI: Cursor Set >> Idle"  # UI: StatusString >> Initializing... UI: Cursor Set >> Busy UI: Start Button >> Connecting UI: StatusString >> Initializing Data Data: Initialize UI: StatusString >> Initializing Core Data Initialize Core Data UI: StatusString >> Initializing User Interface UI: Initialize UI: StatusString >> Initializing Connections Connections: Initialize UI: StatusString >> Query Data System: Query Connections: Status UI: Front Panel State >> Open UI: Cursor Set >> Idle
        # "Initialization Macro\n(This is called once, when the VI starts)"
        n153 = call <vilib>:"Add State(s) to Queue__JKI_lib_State_Machine.vi"("State(s) in Front (\"\")"=w410, "State(s) in (\"\")"=w414) -> ("States Out"=w413:string)  [unwired: 13 in]
      }
      frame "Macro: Exit" {
        # "Exit Macro\n(This is called once, when the VI exits)"
        n154 = Unbundle By Name(w422) -> ("Core.Close Panel on Exit?"=w421:bool)
        n155 = Select(t="UI: Front Panel State >> Close", s=w421, f="") -> (s? t:f=w418:string)
        n156 = call <vilib>:"Add State(s) to Queue__JKI_lib_State_Machine.vi"("State(s) in Front (\"\")"="UI: StatusString >> Closing System... Terminating Connections\nConnections: Terminate\nUI: StatusString >> Closing System... Data Cleanup\nData: Cleanup\nUI: StatusString >> Closing System" ("State(s) in Front (\"\")"), "State(s) in (\"\")"=w418, "State(s) at Back (\"\")"="Exit") -> ("States Out"=w417:string)  [unwired: 12 in]
        n157 = call <vilib>:"Add State(s) to Queue__JKI_lib_State_Machine.vi"("State(s) in Front (\"\")"=w417, "State(s) in (\"\")"=w425) -> ("States Out"=w424:string)  [unwired: 13 in]
      }
      frame "---------- System ----------" {
        # "Template Separator\n(You can make a copy of, or modify, this frame)"
        n158 = call <vilib>:"Add State(s) to Queue__JKI_lib_State_Machine.vi"("State(s) in (\"\")"=w429) -> ("States Out"=w428:string)  [unwired: 14 in]
      }
      frame "System: Transmit" {
        # "Your code here.\n(You can make a copy of, or modify, this frame)"
        n159 = Unbundle By Name(w435) -> ("Connections.Arduino.Connected"=w434:bool, "Connections.Arduino.VISA"=w433:refnum<visa-resource-name>)
        n160 = case shown="True" w434 {
          tunnel: w433 -> [_ w442]
          tunnel: w432 -> [w438 w441]
          tunnel: [w438 w440] -> w430
          tunnel: w431 -> [_ w439]
          frame False {
          }
          frame True {
            n161 = VISA Write(VISA resource name=w442, write buffer=w439, error in (no error)=w441) -> (error out=w440:errorcluster)  [unwired: 2 out]
          }
        }
        n162 = call <vilib>:"Add State(s) to Queue__JKI_lib_State_Machine.vi"("State(s) in (\"\")"=w437) -> ("States Out"=w436:string)  [unwired: 14 in]
      }
      frame "System: Query" {
        # "Your code here.\n(You can make a copy of, or modify, this frame)"
        n163 = Unbundle By Name(w448) -> ("Connections.Arduino.Connected"=w447:bool, "Connections.Arduino.VISA"=w446:refnum<visa-resource-name>)
        n164 = case shown="True" w447 {
          tunnel: w446 -> [_ w455]
          tunnel: w445 -> [w451 w454]
          tunnel: [w451 w453] -> w444
          tunnel: "<FL>" ("Arguments") -> [_ w452]
          frame False {
          }
          frame True {
            n165 = VISA Write(VISA resource name=w455, write buffer=w452, error in (no error)=w454) -> (error out=w453:errorcluster)  [unwired: 2 out]
          }
        }
        n166 = call <vilib>:"Add State(s) to Queue__JKI_lib_State_Machine.vi"("State(s) in (\"\")"=w450) -> ("States Out"=w449:string)  [unwired: 14 in]
      }
      frame "System: Download" {
        # "Your code here.\n(You can make a copy of, or modify, this frame)"
        n167 = property on="File List" class="MCListbox (strict)"() -> ("ItemNames"=w460:string[][], "FocusRow"=w459:i32)  [unwired: 2 in, 2 out]
        n168 = Unbundle By Name(w456) -> ("Connections.Arduino.Connected"=w468:bool, "Connections.Arduino.VISA"=w467:refnum<visa-resource-name>)
        n169 = Index Array(array=w460, index (row)=w459, index (col)=0 ("disabled index (col)")) -> (element=w458:string)
        n170 = Concatenate Strings("<FD" ("string"), w458, ">" ("string")) -> (w461:string)
        n171 = case shown="True" w468 {
          tunnel: w467 -> [_ w482]
          tunnel: w466 -> [w472 w481]
          tunnel: [w472 w480] -> w465
          tunnel: w461 -> [_ w479]
          tunnel: [w471 w478] -> w457
          tunnel: w456 -> [w471 w477]
          frame False {
          }
          frame True {
            n172 = VISA Write(VISA resource name=w482, write buffer=w479, error in (no error)=w481) -> (error out=w480:errorcluster)  [unwired: 2 out]
            n173 = local write "Progress"(u8 0 ("Progress")) -> ()
            n174 = Bundle By Name(cluster=w477, "Files.Downloading"=TRUE) -> (w478:T1)
            n175 = property on="File List" class="MCListbox (strict)"("DisabledEnum"=T5."Disabled" ("Disabled")) -> ()  [unwired: 2 in, 2 out]
            n176 = property on="Progress" class="Slide (strict)"("Visible"=TRUE) -> ()  [unwired: 2 in, 2 out]
          }
        }
        n177 = call <vilib>:"Add State(s) to Queue__JKI_lib_State_Machine.vi"("State(s) in (\"\")"=w470) -> ("States Out"=w469:string)  [unwired: 14 in]
      }
      frame "System: Delete" {
        # "Your code here.\n(You can make a copy of, or modify, this frame)"
        n178 = property on="File List" class="MCListbox (strict)"() -> ("ItemNames"=w488:string[][], "FocusRow"=w487:i32)  [unwired: 2 in, 2 out]
        n179 = Unbundle By Name(w483) -> ("Connections.Arduino.Connected"=w496:bool, "Connections.Arduino.VISA"=w495:refnum<visa-resource-name>)
        n180 = Index Array(array=w488, index (row)=w487, index (col)=0 ("disabled index (col)")) -> (element=w486:string)
        n181 = Match Pattern(string=w486, regular expression=".TXT") -> (before substring=w484:string)  [unwired: 1 in, 3 out]
        n182 = Concatenate Strings("<FR" ("string"), w484, ">" ("string")) -> (w489:string)
        n183 = case shown="True" w496 {
          tunnel: w495 -> [_ w505]
          tunnel: w494 -> [w499 w504]
          tunnel: [w499 w501] -> w493
          tunnel: w489 -> [_ w503]
          frame False {
          }
          frame True {
            n184 = VISA Write(VISA resource name=w505, write buffer=w503, error in (no error)=w504) -> (error out=w502:errorcluster)  [unwired: 2 out]
            n185 = call "Stall Data Flow.vim"("value in"=w502, "milliseconds to wait"=u32 500) -> ("value out"=w501:errorcluster)  [unwired: 1 out]
          }
        }
        n186 = call <vilib>:"Add State(s) to Queue__JKI_lib_State_Machine.vi"("State(s) in (\"\")"=w498) -> ("States Out"=w497:string)  [unwired: 14 in]
      }
      frame "System: Download done" {
        # "Your code here.\n(You can make a copy of, or modify, this frame)"
        n187 = local read "Data Feed"() -> (w506:string)
        n188 = call "Download_Save.vi"("error in (no error)"=w508, "Data Feed"=w506, "DataCluster"=w509) -> ("error out"=w507:errorcluster)  [unwired: 8 in]
        n189 = Bundle By Name(cluster=w509, "Files.Downloading"=FALSE) -> (w514:T1)
        n190 = property on="File List" class="MCListbox (strict)"("DisabledEnum"=T5."Enabled" ("Disabled")) -> ()  [unwired: 2 in, 2 out]
        n191 = local write "Progress"(u8 100 ("Progress")) -> ()
        n192 = property on="Progress" class="Slide (strict)"("Visible"=FALSE) -> ()  [unwired: 2 in, 2 out]
        n193 = call <vilib>:"Add State(s) to Queue__JKI_lib_State_Machine.vi"("State(s) in (\"\")"=w516) -> ("States Out"=w515:string)  [unwired: 14 in]
      }
      frame "---------- Tools ----------" {
        # "Template Separator\n(You can make a copy of, or modify, this frame)"
        n194 = call <vilib>:"Add State(s) to Queue__JKI_lib_State_Machine.vi"("State(s) in (\"\")"=w520) -> ("States Out"=w519:string)  [unwired: 14 in]
      }
    }
  }
